vi "I32Dim_to_umDim.vi"(5 "Offset":dbl format="%#_13g", 6 "-10 to 10V range?":bool, 8 "Max Value [um]":dbl, 11 "Input":i16[](array[numeric])=[0, 0]) -> (2 "x*y":dbl[](array[numeric]))   [LabVIEW 2023]
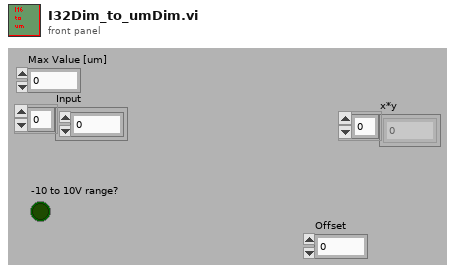
[diagram p1: front panel]
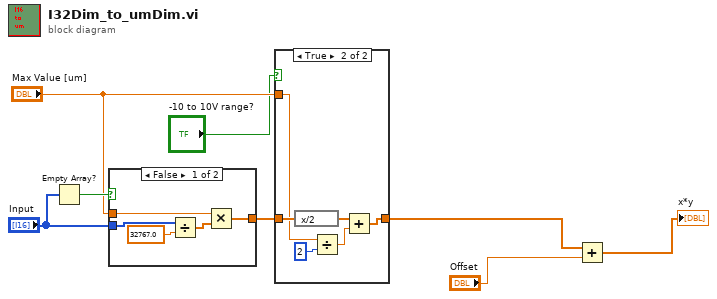
[diagram p0: block diagram]
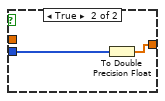
[diagram p3: hidden frame]
diagram:
  n1 = Empty Array?(array="Input") -> (empty?=w7:bool)
  n2 = case shown="False" w7 {
    tunnel: "Input" -> [w11 w15]
    tunnel: [w10 w14] -> w5
    tunnel: "Max Value [um]" -> [w9 _]
    frame False {
      n3 = Divide(x=w11, y=32767.0 ("n")) -> (x/y=w12:dbl[])
      n4 = Multiply(x=w9, y=w12) -> (x*y=w10:dbl[])
    }
    frame True {
      n5 = To Double Precision Float(number=w15) -> (double precision float=w14:dbl[])
    }
  }
  n6 = case shown="True" "-10 to 10V range?" {
    tunnel: [w16 w18] -> w2
    tunnel: w5 -> [w16 w20]
    tunnel: "Max Value [um]" -> [_ w17]
    frame False {
    }
    frame True {
      n7 = expression code="x/2"(w20) -> (w19:dbl[])
      n8 = Divide(x=w17, y=2) -> (x/y=w21:dbl)
      n9 = Add(x=w19, y=w21) -> (x+y=w18:dbl[])
    }
  }
  n10 = Add(x=w2, y="Offset") -> (x+y=→"x*y":dbl[])
